vi "Simple3D.vi"(8 "Angle 2":dbl(knob)=-72.06882847083946 scale=-90.0..90.0, 9 "Angle1":dbl(knob)=-45.83837436417874 scale=-90.0..90.0, 10 "L 2":dbl(slide)=115.0 scale=0.0..200.0, 11 "L 1":dbl(slide)=80.0 scale=0.0..200.0) -> (1 "end effector":cluster{dbl, dbl}={159.01647214211073, 1.9100783062530127} {"?" format="%.1f"; "?" format="%#.1f"})   [LabVIEW 2024]
uses:
  <vilib>/picture/3D Picture Control/Object/Create Object (drawable).vi
  <vilib>/picture/3D Picture Control/Object/Add Object (reference).vi
  <vilib>/picture/3D Picture Control/NI_3D Picture Control.lvlib
panel:
  out "3D Picture":refnum<vi>(3d-picture)
  out "angle":dbl
  out "mag":dbl
  # "A 2"
  # "L1"
  # "L2"
  # "A 1"
  # "mm"
  # "mm"
  # "mm"
  # "mm"
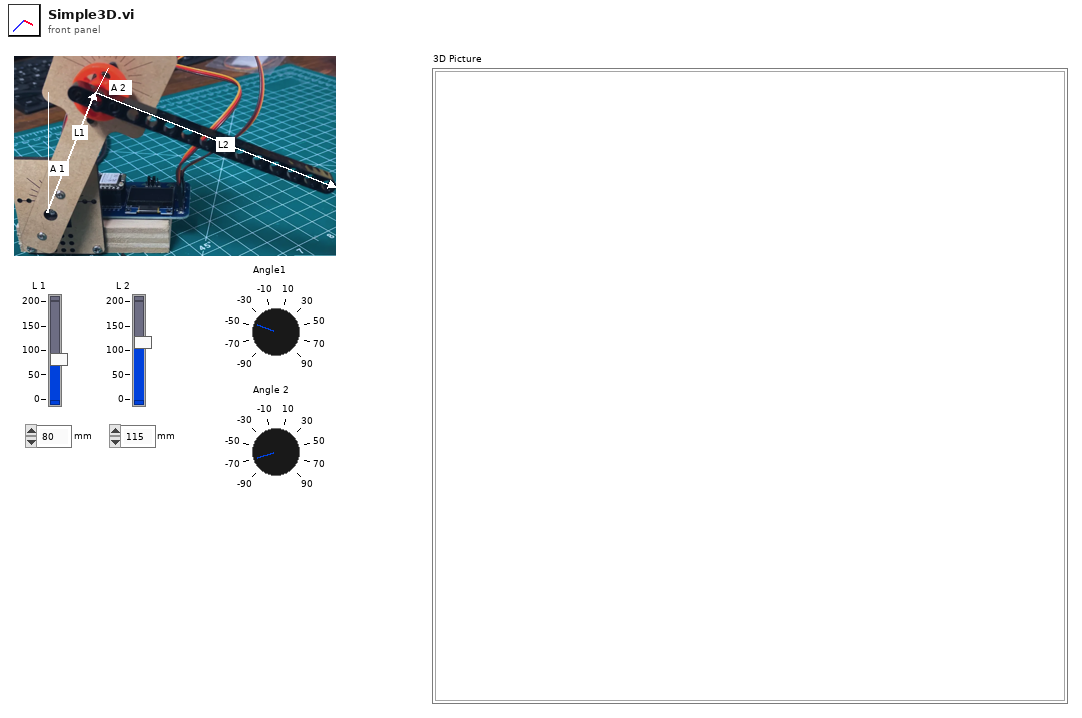
[diagram p1: front panel]
types:
  T1 = cluster{"Red":sgl, "Green":sgl, "Blue":sgl, "Alpha":sgl}
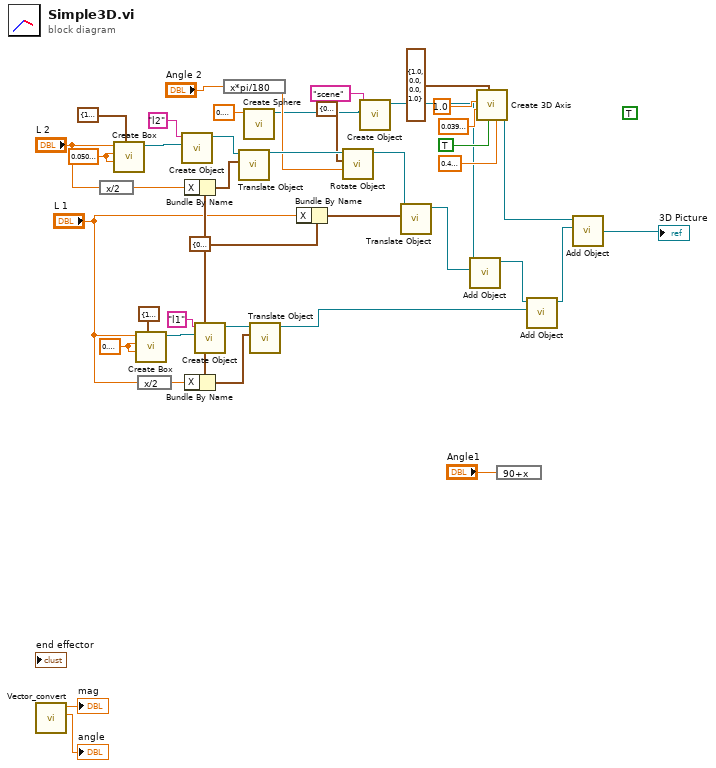
[diagram p0: block diagram]
diagram:
  (unwired) TRUE ("Relative?")
  w19 = cluster{"X":sgl, "Y":sgl, "Z":sgl} {"X"=0.0, "Y"=0.0, "Z"=0.0} ("Translation")
  w23 = sgl 0.05 ("Length Y")
  w39 = sgl 0.1 ("Length Y")
  n1 = call "Vector_convert.vi"() -> ("angle"=→"angle":dbl, "mag"=→"mag":dbl)  [unwired: 10 in]
  n2 = expression code="x/2"("L 2") -> (w28:dbl)
  n3 = call <vilib>:"Create Box.vi"("Color"=T1 {"Red"=1.0, "Green"=1.0, "Blue"=1.0, "Alpha"=1.0}, "Length Z"=w23, "Length Y"=w23, "Length X"="L 2") -> ("New Box Refnum"=w25:refnum<vi>)  [unwired: 6 in, 1 out]
  n4 = call <vilib>:"Create Box.vi"("Color"=T1 {"Red"=1.0, "Green"=1.0, "Blue"=0.0, "Alpha"=1.0}, "Length Z"=w39, "Length Y"=w39, "Length X"="L 1") -> ("New Box Refnum"=w37:refnum<vi>)  [unwired: 6 in, 1 out]
  n5 = expression code="x/2"("L 1") -> (w30:dbl)
  n6 = call-poly <vilib>:"Create Object.vi"("Geometry"=w25, "Name"="l2") -> ("Scene:New Object"=w27:refnum<vi>)  [unwired: 8 in, 1 out]
  n7 = Bundle By Name(cluster=w19, "X"=w28) -> (w20:cluster{"X":sgl, "Y":sgl, "Z":sgl})
  n8 = Bundle By Name(cluster=w19, "X"=w30) -> (w21:cluster{"X":sgl, "Y":sgl, "Z":sgl})
  n9 = call-poly <vilib>:"Create Object.vi"("Geometry"=w37, "Name"="l1") -> ("Scene:New Object"=w3:refnum<vi>)  [unwired: 8 in, 1 out]
  n10 = expression code="x*pi/180"("Angle 2") -> (w13:dbl)
  n11 = call <vilib>:"Translate Object.vi"("Translation"=w20, "Scene.Object In"=w27) -> ("Scene.Object Out"=w16:refnum<vi>)  [unwired: 8 in, 1 out]
  n12 = call <vilib>:"Create Sphere.vi"("Radius"=sgl 0.1) -> ("New Sphere Refnum"=w8:refnum<vi>)  [unwired: 9 in, 1 out]
  n13 = call <vilib>:"Translate Object.vi"("Translation"=w21, "Scene.Object In"=w3) -> ("Scene.Object Out"=w1:refnum<vi>)  [unwired: 8 in, 1 out]
  n14 = Bundle By Name(cluster=w19, "X"="L 1") -> (w17:cluster{"X":sgl, "Y":sgl, "Z":sgl})
  n15 = call <vilib>:"Rotate Object.vi"("Angle"=w13, "Axis"=cluster{"X":sgl, "Y":sgl, "Z":sgl} {"X"=0.0, "Y"=0.0, "Z"=1.0}, "Scene.Object In"=w16) -> ("Scene.Object Out"=w12:refnum<vi>)  [unwired: 7 in, 1 out]
  n16 = call-poly <vilib>:"Create Object.vi"("Geometry"=w8, "Name"="scene") -> ("Scene:New Object"=w9:refnum<vi>)  [unwired: 8 in, 1 out]
  n17 = call <vilib>:"Translate Object.vi"("Translation"=w17, "Scene.Object In"=w12) -> ("Scene.Object Out"=w11:refnum<vi>)  [unwired: 8 in, 1 out]
  n18 = call-poly <vilib>:"Add Object.vi"("New Object In"=w11, "Scene Object In"=w9) -> ("Scene Object Out"=w4:refnum<vi>)  [unwired: 7 in, 2 out]
  n19 = call <vilib>:"Create 3D Axis.vi"("Character Size"=sgl 0.4, "Axis label?"=TRUE, "Color"=T1 {"Red"=1.0, "Green"=0.0, "Blue"=0.0, "Alpha"=1.0}, "Radius"=sgl 0.04, "Length"=sgl 1.0) -> ("New Object Refnum"=w6:refnum<vi>)  [unwired: 5 in, 1 out]
  n20 = expression code="90+x"("Angle1") -> ()  [unwired: 1 out]
  n21 = call-poly <vilib>:"Add Object.vi"("New Object In"=w1, "Scene Object In"=w4) -> ("Scene Object Out"=w2:refnum<vi>)  [unwired: 7 in, 2 out]
  n22 = call-poly <vilib>:"Add Object.vi"("New Object In"=w2, "Scene Object In"=w6) -> ("Scene Object Out"=→"3D Picture":refnum<vi>)  [unwired: 7 in, 2 out]
